vi "Recieve Response with Result.vi"(4 "Finished":bool=TRUE, 6 "Result":refnum<class "Mag Lab Result.lvclass">, 8 "error in (no error)":errorcluster, 9 "Requestor":string, 10 "Requestee":string, 11 "Compound Measurement in":refnum<class "Compound Measurement.lvclass">) -> (0 "error out":errorcluster, 3 "Compound Measurement out":refnum<class "Compound Measurement.lvclass">)   [LabVIEW 2015, in "Compound Measurement.lvclass"]
uses:
  Compound Measurement.lvclass
  Mag Lab Result/Mag Lab Result.lvclass
  Mag Lab Root/Mag Lab Root.lvclass/Mag Lab Root.ctl
  Compound Measurement.lvclass/Compound Measurement.ctl
  Mag Lab Result/Mag Lab Result.lvclass/Mag Lab Result.ctl
  <vilib>/ActorFramework/Actor/Actor.lvclass/Actor.ctl
  <vilib>/ActorFramework/Message Enqueuer/Message Enqueuer.lvclass/Message Enqueuer.ctl
  Mag Lab Root Messages/Recieve Response with Result Msg/Recieve Response with Result Msg.lvclass/Recieve Response with Result Msg.ctl
  Mag Lab Result/Read Sets pace.vi
  Mag Lab Result/Read Next time.vi
  Mag Lab Root/Read Original requestor.vi
  Mag Lab Root/Read Name.vi
  Mag Lab Root/Read Synchronous operation.vi
  <vilib>/ActorFramework/Message Enqueuer/Init from Existing Queue.vi
  <vilib>/ActorFramework/Message Enqueuer/Enqueue.vi
  <vilib>/ActorFramework/Message Priority Queue/Priority Enqueue.vi
  <vilib>/ActorFramework/Message Enqueuer/Message Enqueuer.lvclass
  Mag Lab Root Messages/Recieve Response with Result Msg/Recieve Response with Result Msg.lvclass
  <vilib>/ActorFramework/Actor/Actor.lvclass
  Mag Lab Error Handler/Mag Lab Error Handler.lvclass
  Mag Lab Root/Mag Lab Root.lvclass
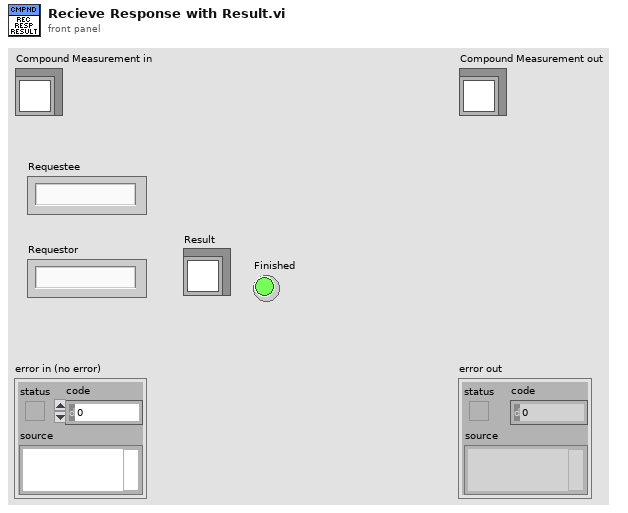
[diagram p1: front panel]
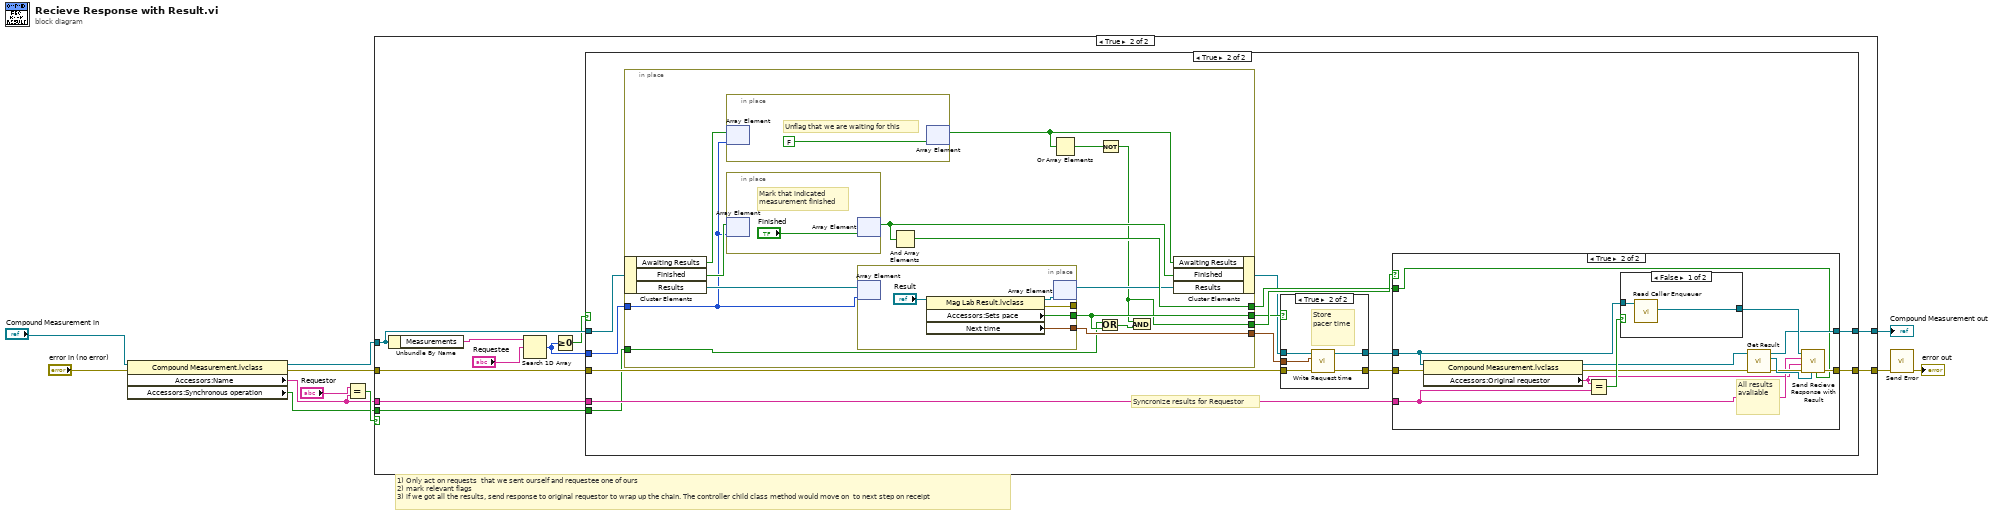
[diagram p0: block diagram]
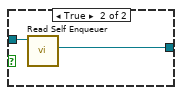
[diagram p6: hidden frame]
diagram:
  # "1) Only act on requests  that we sent ourself and requestee one of ours\n2) mark relevant flags \n3) if we got all the results, send response to original requestor to wrap up the chain. The controller child class method would move on  to next step on receipt"
  n1 = property class="Compound Measurement.lvclass"(reference="Compound Measurement in", error in="error in (no error)") -> (reference out=w4:refnum<class "Compound Measurement.lvclass">, error out=w2:errorcluster, "Accessors:Name"=w5:string, "Accessors:Synchronous operation"=w1:bool)
  n2 = Equal?(x="Requestor", y=w5) -> (x = y?=w11:bool)
  n3 = case shown="True" w11 {
    tunnel: w4 -> [w13 w21]
    tunnel: [w13 w19] -> w10
    tunnel: w5 -> [_ w17]
    tunnel: [w12 w16] -> w8
    tunnel: w2 -> [w12 w15]
    tunnel: w1 -> [_ w14]
    frame False {
    }
    frame True {
      n4 = Unbundle By Name(w21) -> ("Measurements"=w23:string[])
      n5 = Search 1D Array(1D array=w23, element="Requestee") -> (index of element=w20:i32)  [unwired: 1 in]
      n6 = Greater Or Equal To 0?(x=w20) -> (x >= 0?=w18:bool)
      n7 = case shown="True" w18 {
        tunnel: w21 -> [w25 w39]
        tunnel: w20 -> [_ w38]
        tunnel: [w25 w35] -> w19
        tunnel: w17 -> [_ w36]
        tunnel: [w24 w34] -> w16
        tunnel: w15 -> [w24 w31]
        tunnel: w14 -> [_ w28]
        frame False {
        }
        frame True {
          # "Syncronize results for Requestor"
          n8 = in-place {
            in-place-border: w38 -> [w73]
            in-place-border: [w66] -> w37
            in-place-border: [w75] -> w33
            in-place-border: [w69] -> w32
            in-place-border: [w71] -> w29
            in-place-border: w28 -> [w68]
            n9 = in-place-cluster #1(w39) -> ("Awaiting Results"=w79:bool[], "Finished"=w77:bool[], "Results"=w74:refnum<class "Mag Lab Result.lvclass">[])
            n10 = in-place {
              # "Unflag that we are waiting for this"
              n11 = in-place-array #2(w79, w73) -> ()  [unwired: 1 out]
              n12 = in-place-array #2(FALSE ("new element/subarray")) -> (w78:bool[])  [unwired: 1 out]
            }
            n13 = in-place {
              # "Mark that indicated \nmeasurement finished"
              n14 = in-place-array #3(w77, w73) -> ()  [unwired: 1 out]
              n15 = in-place-array #3("Finished") -> (w76:bool[])  [unwired: 1 out]
            }
            n16 = in-place {
              in-place-border: [w82] -> _
              in-place-border: [w81] -> w69
              in-place-border: [w80] -> w71
              n17 = in-place-array #4(w74, w73) -> ()  [unwired: 1 out]
              n18 = property class="Mag Lab Result.lvclass"(reference="Result") -> (reference out=w83:refnum<class "Mag Lab Result.lvclass">, error out=w82:errorcluster, "Accessors:Sets pace"=w81:bool, "Next time"=w80:timestamp)  [unwired: 1 in]
              n19 = in-place-array #4(w83) -> (w72:refnum<class "Mag Lab Result.lvclass">[])  [unwired: 1 out]
            }
            n20 = And Array Elements(Boolean array=w76) -> (logical AND=w75:bool)
            n21 = Or Array Elements(Boolean array=w78) -> (logical OR=w70:bool)
            n22 = Or(x=w68, y=w69) -> (x .or. y?=w67:bool)
            n23 = Not(x=w70) -> (.not. x?=w66:bool)
            n24 = And(x=w66, y=w67) -> ()  [unwired: 1 out]
            n25 = in-place-cluster #1("Awaiting Results"=w78, "Finished"=w76, "Results"=w72) -> (w27:refnum<class "Compound Measurement.lvclass">)
          }
          n26 = case shown="True" w32 {
            tunnel: w31 -> [w41 w46]
            tunnel: [w41 w45] -> w30
            tunnel: w29 -> [_ w44]
            tunnel: w27 -> [w40 w42]
            tunnel: [w40 w43] -> w26
            frame False {
            }
            frame True {
              # "Store  pacer time"
              n27 = call "Write Request time.vi"("error in (no error)"=w46, "Request time"=w44, "Mag Lab Root in"=w42) -> ("error out"=w45:errorcluster, "Mag Lab Root out"=w43:refnum<class "Compound Measurement.lvclass">)  [unwired: 7 in]
            }
          }
          n28 = case shown="True" w37 {
            tunnel: w26 -> [w48 w60]
            tunnel: w36 -> [_ w54]
            tunnel: [w48 w56] -> w35
            tunnel: [w47 w57] -> w34
            tunnel: w30 -> [w47 w50]
            tunnel: w33 -> [_ w55]
            frame False {
            }
            frame True {
              # "All results avaliable"
              n29 = property class="Compound Measurement.lvclass"(reference=w60, error in=w50) -> (reference out=w52:refnum<class "Compound Measurement.lvclass">, error out=w49:errorcluster, "Accessors:Original requestor"=w51:string)
              n30 = Equal?(x=w51, y=w54) -> (x = y?=w53:bool)
              n31 = case shown="False" w53 {
                tunnel: [w63 w64] -> w61
                tunnel: w60 -> [w62 w65]
                frame False {
                  n32 = call <vilib>:"Read Caller Enqueuer.vi"("Actor"=w62) -> ("Caller Enqueuer"=w63:refnum<class "Message Enqueuer.lvclass">)  [unwired: 10 in]
                }
                frame True {
                  n33 = call <vilib>:"Read Self Enqueuer.vi"("Actor"=w65) -> ("Self Enqueuer"=w64:refnum<class "Message Enqueuer.lvclass">)  [unwired: 10 in]
                }
              }
              n34 = call-dynamic "Get Result.vi"("error in (no error)"=w49, "Mag Lab Root in"=w52) -> ("error out"=w58:errorcluster, "Result"=w59:refnum<class "Mag Lab Result.lvclass">, "Mag Lab Root out"=w56:refnum<class "Compound Measurement.lvclass">)  [unwired: 7 in]
              n35 = call "Send Recieve Response with Result.vi"("Finished"=w55, "Result"=w59, "error in (no error)"=w58, "Requestor"=w51, "Requestee"=w54, "Message Enqueuer"=w61) -> ("error out"=w57:errorcluster)  [unwired: 4 in, 1 out]
            }
          }
        }
      }
    }
  }
  "Compound Measurement out" <- w10
  n36 = call "Send Error.vi"("error in (no error)"=w8) -> ("error out"=→"error out":errorcluster)  [unwired: 9 in, 1 out]
